vi "Close.vi"(8 "error in":errorcluster, 11 "MSS in":refnum<class "MSS.lvclass">) -> (0 "error out":errorcluster, 3 "MSS out":refnum<class "MSS.lvclass">)   [LabVIEW 2023, in "HAL.lvlib" / "MSS.lvclass"]
uses:
  MSS.lvclass
  MSS.lvclass/MSS.ctl
  Instrument/Instrument.lvclass
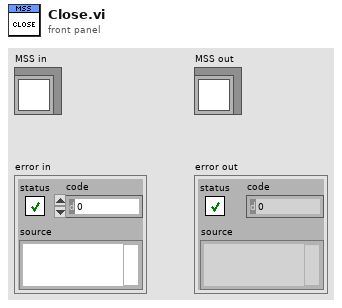
[diagram p1: front panel]
types:
  T1 = map{string, cluster{"Instrument":refnum<class "Instrument.lvclass">, "Ref Count":i16}}
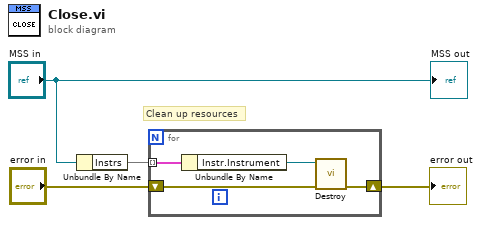
[diagram p0: block diagram]
diagram:
  # "Clean up resources"
  n1 = Unbundle By Name("MSS in") -> ("Instrs"=w4:T1)
  n2 = for {
    tunnel: w4 -> [w8] mode=indexing
    shift-right: [w6] -> w2
    shift-left: "error in" -> [w7]
    n3 = Unbundle By Name(w8) -> ("Instr.Instrument"=w5:refnum<class "Instrument.lvclass">)
    n4 = call-dynamic "Destroy.vi"("Error In"=w7, "reference in"=w5) -> ("Error Out"=w6:errorcluster)  [unwired: 8 in, 1 out]
  }
  "error out" <- w2
  "MSS out" <- "MSS in"
